vi "Do.vi"(8 "error in (no error)":errorcluster, 9 "Events":refnum<class "Events.lvclass">, 10 "Message Loop Data in":T1, 11 "IInternalRequest in":refnum<class "InvocationHandler JSON.lvclass">) -> (0 "error out":errorcluster, 2 "Message Loop Data out":T1, 3 "IInternalRequest out":refnum<class "InvocationHandler JSON.lvclass">)   [LabVIEW 2020, in "wamplv.lvlib" / "InvocationHandler JSON.lvclass"]
uses:
  InvocationHandler JSON.lvclass
  InvocationHandler JSON.lvclass/InvocationHandler JSON.ctl
  Invocation Request ID/Invocation Request ID.lvclass
  WAMP Client/API/TypeDefs/INVOCATION payload.ctl
  WAMP Client/WAMP Client.lvclass
  Events/JsonEvents/JsonEvents.lvclass
  SerialisedMessages/JSONMessage/WampMessage JSON.lvclass
  Utils/Utils.lvclass
  WAMP Client/Private/TypeDef/Publish Requests Map.ctl
  wamplv.lvlib
  WAMP Client/Private/TypeDef/Endpoint Data.ctl
  Call/ICallRequest/ICallRequest.lvclass
  WAMP Client/Private/TypeDef/CALL Request Map.ctl
  WAMP Client/Private/TypeDef/SUBSCRIBE Requests Map.ctl
  WAMP Client/Private/TypeDef/Subscriptions Map.ctl
  WAMP Client/Private/TypeDef/Unsubscribe Requests Map.ctl
  WAMP Client/Private/TypeDef/Unregister requests map.ctl
  WAMP Client/Private/TypeDef/Message Loop Data.ctl
  Events/EventsParent/Events.lvclass
  Subscribe/ISubscribe/ISubscribe.lvclass
  Publish/IPublish/IPublish.lvclass
  Message loop classes/Subscription details/SubscriptionDetailsParent/SubscriptionDetailsParent.lvclass
  Unsubscribe/IUnsubscribe/IUnsubscribe.lvclass
  Register/IRegister/IRegister.lvclass
  Unregister/IUnregister/IUnregister.lvclass
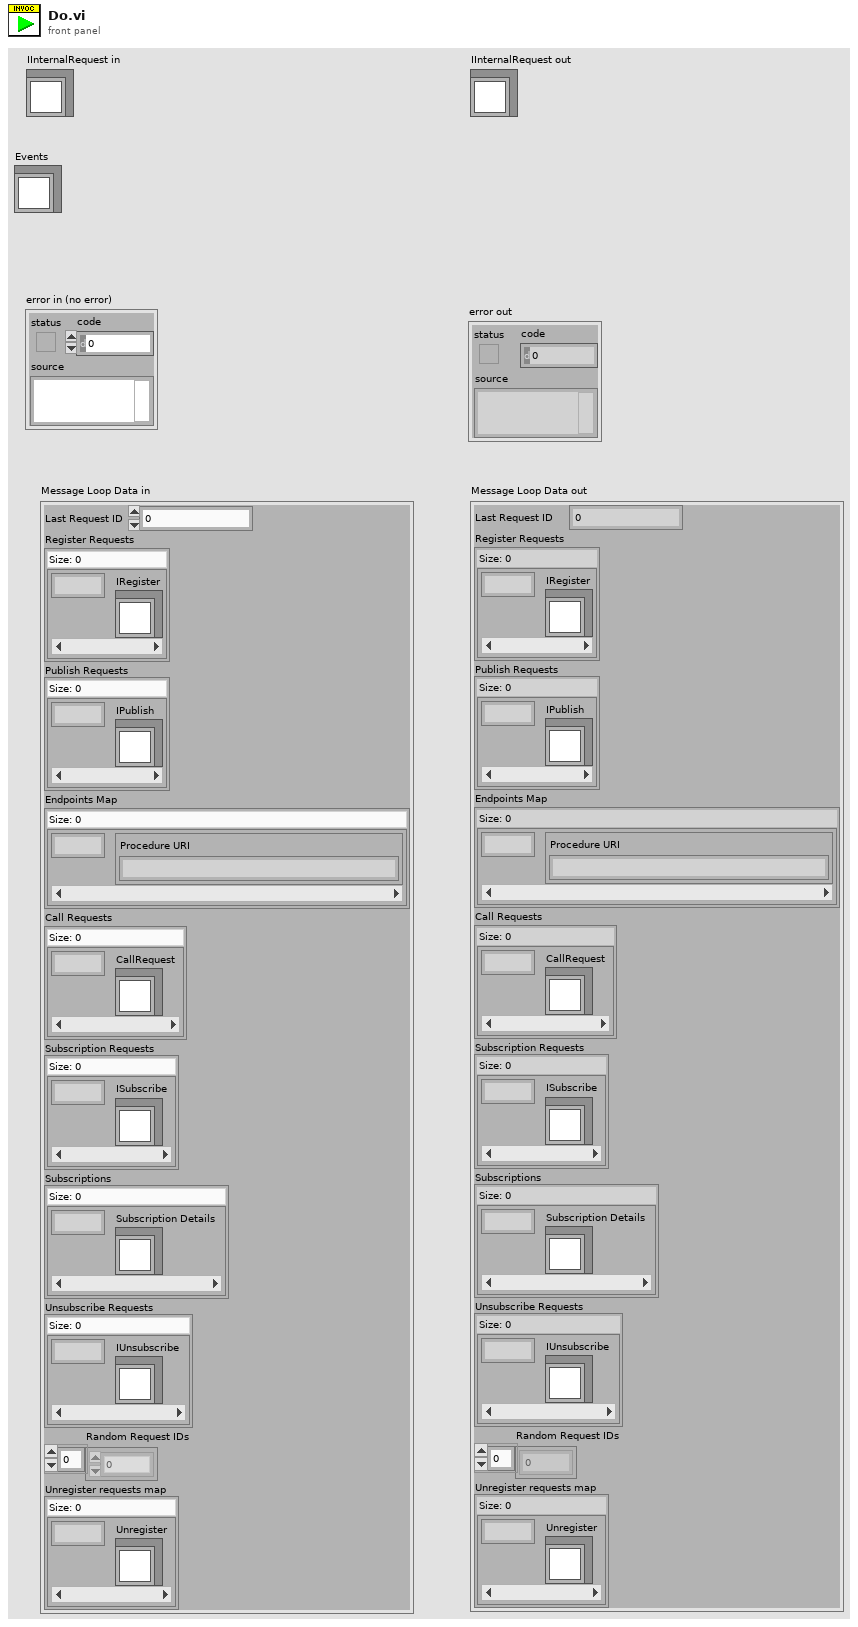
[diagram p1: front panel]
types:
  T1 = typedef "wamplv.lvlib/Message Loop Data.ctl" = cluster{"Last Request ID":u64, "Register Requests":map{u64, refnum<class "IRegister.lvclass">}, "Publish Requests":T2, "Endpoints Map":map{u64, T3}, "Call Requests":T4, "Subscription Requests":T5, "Subscriptions":T6, "Unsubscribe Requests":T7, "Random Request IDs":u64[], "Unregister requests map":T8}
  T2 = typedef "wamplv.lvlib/Publish Requests Map.ctl" = map{u64, refnum<class "IPublish.lvclass">}
  T3 = typedef "wamplv.lvlib/Endpoint Data.ctl" = cluster{"Procedure URI":string}
  T4 = typedef "wamplv.lvlib/CALL Request Map.ctl" = map{u64, refnum<class "ICallRequest.lvclass">}
  T5 = typedef "wamplv.lvlib/SUBSCRIBE Requests Map.ctl" = map{u64, refnum<class "ISubscribe.lvclass">}
  T6 = typedef "wamplv.lvlib/Subscriptions Map.ctl" = map{u64, refnum<class "SubscriptionDetailsParent.lvclass">}
  T7 = typedef "wamplv.lvlib/Unsubscribe Requests Map.ctl" = map{u64, refnum<class "IUnsubscribe.lvclass">}
  T8 = typedef "wamplv.lvlib/Unregister requests map.ctl" = map{u64, refnum<class "IUnregister.lvclass">}
  T9 = typedef "wamplv.lvlib/WAMP Client.lvclass/INVOCATION payload.ctl" = cluster{"Arguments":string, "ArgumentKw":string, "Procedure URI":string, "Details":string, "Registration ID":u64, "Invocation Request ID":refnum<class "Invocation Request ID.lvclass">}
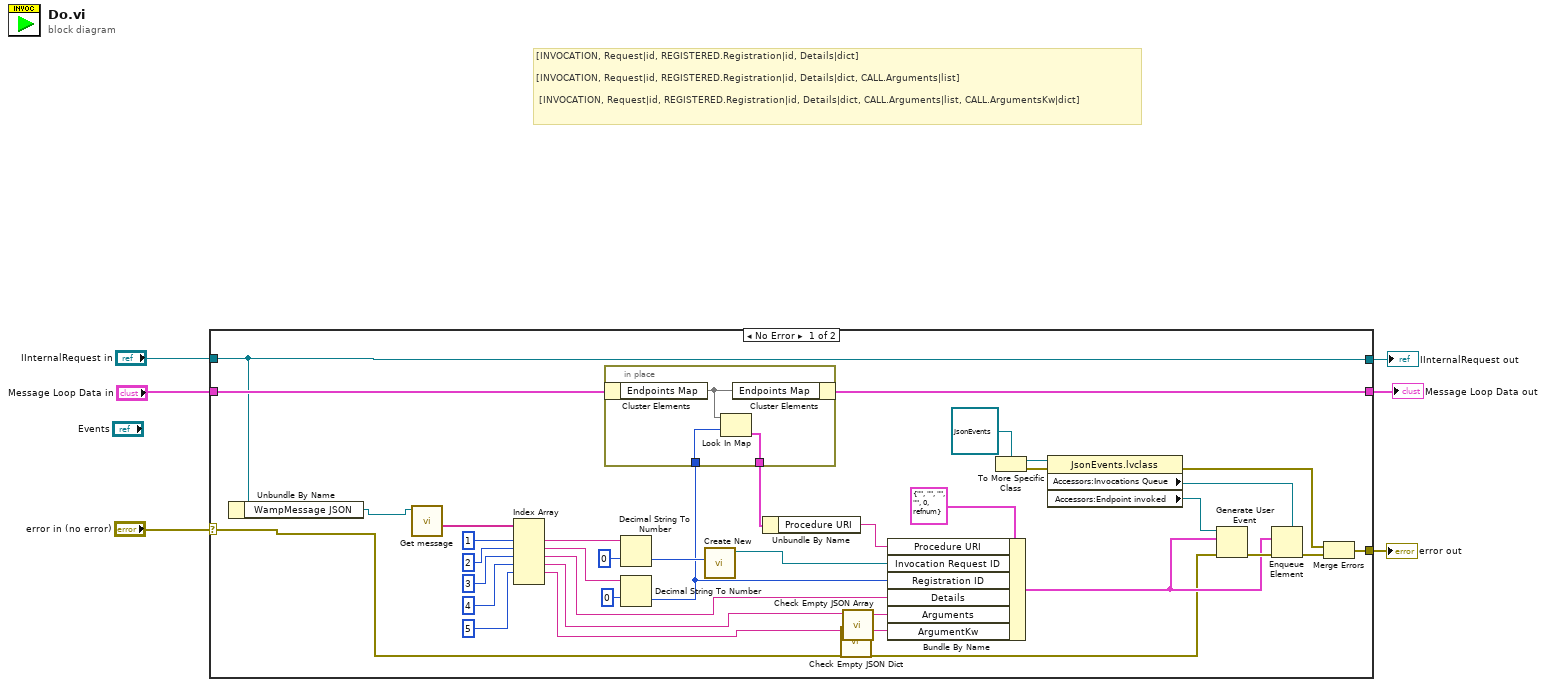
[diagram p0: block diagram]
diagram:
  # "[INVOCATION, Request|id, REGISTERED.Registration|id, Details|dict]\n\n[INVOCATION, Request|id, REGISTERED.Registration|id, Details|dict, CALL.Arguments|list]\n\n [INVOCATION, Request|id, REGISTERED.Registration|id, Details|dict, CALL.Arguments|list, CALL.ArgumentsKw|dict]"
  n1 = case shown="No Error" "error in (no error)" {
    selector: "error in (no error)" -> [w7 w46]
    tunnel: "Message Loop Data in" -> [w25 w47]
    tunnel: [w24 w47] -> w5
    tunnel: "IInternalRequest in" -> [w8 w48]
    tunnel: [w8 w48] -> w3
    tunnel: [w22 w46] -> w1
    frame No Error {
      n2 = Unbundle By Name(w8) -> ("WampMessage JSON"=w9:refnum<class "WampMessage JSON.lvclass">)
      n3 = call "Get message.vi"("JSONMessage in"=w9) -> ("<JSON>Elements"=w23:string[])  [unwired: 8 in, 2 out]
      n4 = Index Array(array=w23, index #1=1 ("index"), index #2=2 ("index"), index #3=3 ("index"), index #4=4 ("index"), index #5=5 ("index")) -> (element #1=w42:string, element #2=w17:string, element #3=w16:string, element #4=w12:string, element #5=w10:string)  [unwired: 1 in, 1 out]
      n5 = Decimal String To Number(string=w42, default (0L)=u64 0) -> (number=w33:u64)  [unwired: 1 in, 1 out]
      n6 = Decimal String To Number(string=w17, default (0L)=u64 0) -> (number=w31:u64)  [unwired: 1 in, 1 out]
      n7 = in-place {
        in-place-border: [w44] -> w38
        in-place-border: w31 -> [w45]
        n8 = in-place-cluster #1(w25) -> ("Endpoints Map"=w43:map{u64, T3})
        n9 = Look In Map(map=w43, key=w45) -> (value=w44:T3)  [unwired: 1 in, 1 out]
        n10 = in-place-cluster #1("Endpoints Map"=w43) -> (w24:T1)
      }
      n11 = call "Create New.vi"("Invocation Request ID"=w33) -> ("Invocation Request out"=w32:refnum<class "Invocation Request ID.lvclass">)  [unwired: 9 in, 1 out]
      n12 = Unbundle By Name(w38) -> ("Procedure URI"=w37:string)
      n13 = call "Check Empty JSON Dict.vi"("JSON in"=w10) -> ("JSON out"=w11:string)  [unwired: 10 in]
      n14 = call "Check Empty JSON Array.vi"("JSON in"=w12) -> ("JSON out"=w13:string)  [unwired: 10 in]
      n15 = Bundle By Name(cluster=T9 {"Arguments"="", "ArgumentKw"="", "Procedure URI"="", "Details"="", "Registration ID"=0, "Invocation Request ID"=refnum} ("INVOCATION payload"), "Procedure URI"=w37, "Invocation Request ID"=w32, "Registration ID"=w31, "Details"=w16, "Arguments"=w13, "ArgumentKw"=w11) -> (w34:T9)
      n16 = To More Specific Class(target class=refnum<class "JsonEvents.lvclass"> refnum ("wamplv.lvlib:JsonEvents.lvclass")) -> (specific class reference=w29:refnum<class "JsonEvents.lvclass">, error out=w28:errorcluster)  [unwired: 2 in]
      n17 = property class="JsonEvents.lvclass"(reference=w29, error in=w28) -> (error out=w21:errorcluster, "Accessors:Invocations Queue"=w26:refnum<queue>, "Accessors:Endpoint invoked "=w27:refnum<user-event>)  [unwired: 1 out]
      n18 = Generate User Event(user event=w27, event data cluster=w34, error in=w7) -> (error out=w35:errorcluster)  [unwired: 1 in, 1 out]
      n19 = Enqueue Element(queue=w26, element=w34, error in (no error)=w35) -> (error out=w20:errorcluster)  [unwired: 1 in, 2 out]
      n20 = Merge Errors(w21, w20) -> (w22:errorcluster)
    }
    frame Error {
    }
  }
  "error out" <- w1
  "IInternalRequest out" <- w3
  "Message Loop Data out" <- w5
